vi "Get Curr and Volt.vi"(0 "Keysight in":refnum<class "Keysight.lvclass">, 11 "error in (no error)":errorcluster) -> (4 "Keysight out":refnum<class "Keysight.lvclass">, 6 "Voltage":dbl, 8 "Current":dbl, 10 "Output?":bool, 15 "error out":errorcluster)   [LabVIEW 2020, in "PS.lvlib" / "Keysight.lvclass"]
uses:
  Keysight.lvclass
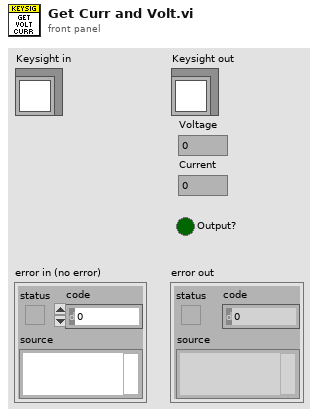
[diagram p1: front panel]
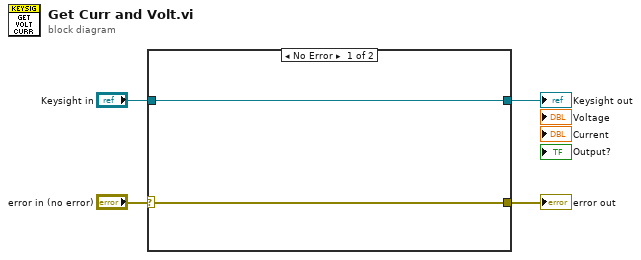
[diagram p0: block diagram]
diagram:
  n1 = case shown="No Error" "error in (no error)" {
    selector: "error in (no error)" -> [w6 w7]
    tunnel: [w5 w8] -> w3
    tunnel: "Keysight in" -> [w5 w8]
    tunnel: [w6 w7] -> w1
    frame No Error {
    }
    frame Error {
    }
  }
  "error out" <- w1
  "Keysight out" <- w3
